vi "HFRR ADV v05 new software.vi"() -> ()   [LabVIEW 2025] (continued)
                  n3128 = property on="Air Temperature  ( °C )" class="XYGraph (strict)"("Y Scale.Name Label.Text"=w4162) -> ()  [unwired: 2 in, 2 out]
                }
                frame 82 {
                  n3129 = local write "S 84"(w4163) -> ()
                }
                frame 83 {
                  n3130 = local write "S 85"(w4164) -> ()
                }
                frame 84 {
                  n3131 = local write "S 86"(w4165) -> ()
                }
                frame 85 {
                  n3132 = local write "S 87"(w4166) -> ()
                }
                frame 86 {
                  n3133 = local write "S 88"(w4167) -> ()
                }
                frame 87 {
                }
                frame 88 {
                  n3134 = local write "S 90"(w4169) -> ()
                }
                frame 89 {
                  n3135 = local write "S 91"(w4170) -> ()
                }
                frame 90 {
                  n3136 = local write "S 92"(w4171) -> ()
                }
                frame 91 {
                  n3137 = local write "S 93"(w4172) -> ()
                }
                frame 92 {
                  n3138 = local write "S 94"(w4173) -> ()
                }
                frame 93 {
                  n3139 = local write "S 95"(w4174) -> ()
                }
                frame 94 {
                  n3140 = local write "S 96"(w4175) -> ()
                }
                frame 95 {
                  n3141 = local write "S 97"(w4176) -> ()
                }
                frame 96 {
                  n3142 = local write "S 98"(w4177) -> ()
                }
                frame 97 {
                  n3143 = local write "S 99"(w4178) -> ()
                }
                frame 98 {
                  n3144 = local write "S 100"(w4179) -> ()
                }
                frame 99 {
                  n3145 = local write "S 101"(w4180) -> ()
                }
                frame 100 {
                  n3146 = local write "S 102"(w4181) -> ()
                }
                frame 101 {
                  n3147 = local write "S 103"(w4182) -> ()
                }
                frame 102 {
                  n3148 = local write "S 104"(w4183) -> ()
                }
                frame 103 {
                  n3149 = local write "S 105"(w4184) -> ()
                }
                frame 104 {
                  n3150 = local write "S 106"(w4185) -> ()
                }
                frame 105 {
                }
                frame 106 {
                  n3151 = property on="OK Button 17" class="Bool (strict)"("Boolean Text.Text"=w4186) -> ()  [unwired: 2 in, 2 out]
                }
                frame 107 {
                  n3152 = property on="OK Button 16" class="Bool (strict)"("Boolean Text.Text"=w4187) -> ()  [unwired: 2 in, 2 out]
                }
                frame 108 {
                  n3153 = property on="TITTLE" class="Str"("Caption.Text"=w4188) -> ()  [unwired: 2 in, 2 out]
                }
                frame 109 {
                  "String 30" <- w4189
                }
                frame 110 {
                  n3154 = property on="Test Date" class="Str"("Caption.Text"=w4190) -> ()  [unwired: 2 in, 2 out]
                  "String 31" <- w4190
                }
                frame 111 {
                  n3155 = property on="Sample ID" class="Str"("Caption.Text"=w4191) -> ()  [unwired: 2 in, 2 out]
                  "String 32" <- w4191
                }
                frame 112 {
                  n3156 = property on="Tested by" class="Str"("Caption.Text"=w4192) -> ()  [unwired: 2 in, 2 out]
                  "String 33" <- w4192
                }
                frame 113 {
                  n3157 = property on="System Configured Printers 2" class="Arr (strict)"("Caption.Text"=w4193) -> ()  [unwired: 2 in, 2 out]
                }
                frame 114 {
                  n3158 = property on="Selected Printer" class="Str"("Caption.Text"=w4194) -> ()  [unwired: 2 in, 2 out]
                }
                frame 115 {
                  n3159 = property on="Select Printer 3" class="DigNum (strict)"("Caption.Text"=w4195) -> ()  [unwired: 2 in, 2 out]
                }
                frame 116 {
                  n3160 = property on="Print" class="Bool (strict)"("Boolean Text.Text"=w4196) -> ()  [unwired: 2 in, 2 out]
                }
                frame 117 {
                  "String 41" <- w4197
                }
                frame 118 {
                  n3161 = property on="tested by" class="Str"("Caption.Text"=w4198) -> ()  [unwired: 2 in, 2 out]
                }
                frame 119 {
                }
                frame 120 {
                  n3162 = property on="Export" class="Bool (strict)"("Boolean Text.Text"=w4199) -> ()  [unwired: 2 in, 2 out]
                }
                frame 121 {
                  n3163 = property on="TEMP INTERCEPT:" class="DigNum (strict)"("Caption.Text"=w4200) -> ()  [unwired: 2 in, 2 out]
                }
                frame 122 {
                  n3164 = property on="AIR TEMP INTERCEPT:" class="DigNum (strict)"("Caption.Text"=w4201) -> ()  [unwired: 2 in, 2 out]
                }
                frame 123 {
                  n3165 = property on="Select File Type" class="Enum (strict)"("Caption.Text"=w4202) -> ()  [unwired: 2 in, 2 out]
                }
                frame 124 {
                  n3166 = property on="s.NO" class="Str"("Caption.Text"=w4203) -> ()  [unwired: 2 in, 2 out]
                  "String 45" <- w4203
                }
                frame 125 {
                  n3167 = property on="trip1 8" class="Bool (strict)"("Boolean Text.Text"=w4204) -> ()  [unwired: 2 in, 2 out]
                }
                frame 126, Default {
                }
              }
            }
          }
          frame #1 {
            w4212 = TRUE ("Visible")
            n3168 = local read "S 91"() -> (w4229:string)
            n3169 = local read "S 90"() -> (w4228:string)
            n3170 = local read "S 88"() -> (w4227:string)
            n3171 = property on="File Path" class="Path"("Caption.Text"=w4228) -> ()  [unwired: 2 in, 2 out]
            n3172 = property on="SrvM CP" class="Bool (strict)"("Boolean Text.Text"=w4227) -> ()  [unwired: 2 in, 2 out]
            n3173 = local read "S 71"() -> (w4222:string)
            n3174 = local read "S 86"() -> (w4224:string)
            n3175 = local read "S 85"() -> (w4225:string)
            n3176 = local read "S 87"() -> (w4223:string)
            n3177 = local read "S 84"() -> (w4226:string)
            n3178 = local read "S 103"() -> (w4211:string)
            n3179 = local read "S 104"() -> (w4210:string)
            n3180 = property on="ENTER THE NEW PASSWORD" class="Str"("Caption.Text"=w4223) -> ()  [unwired: 2 in, 2 out]
            n3181 = property on="Password" class="Str"("Caption.Text"=w4225) -> ()  [unwired: 2 in, 2 out]
            n3182 = property on="ENTER CURRENT PASSWORD" class="Str"("Caption.Text"=w4224) -> ()  [unwired: 2 in, 2 out]
            n3183 = property on="EDIT" class="Bool (strict)"("Boolean Text.Text"=w4222) -> ()  [unwired: 2 in, 2 out]
            n3184 = property on="SAVE" class="Bool (strict)"("Boolean Text.Text"=w4226) -> ()  [unwired: 2 in, 2 out]
            n3185 = Build Array(w4211, w4210) -> (w4209:string[])
            n3186 = property on="Heater Button" class="Bool (strict)"("Strings [4]"=w4209) -> ()  [unwired: 2 in, 2 out]
            n3187 = property on="CH-HUMIDITY WET" class="DigNum (strict)"("Caption.Size to Text?"=w4212) -> ()  [unwired: 2 in, 2 out]
            n3188 = property on="CH-HUMIDITY DRY" class="DigNum (strict)"("Caption.Size to Text?"=w4212) -> ()  [unwired: 2 in, 2 out]
            n3189 = property on="CH-POWER -" class="DigNum (strict)"("Caption.Size to Text?"=w4212) -> ()  [unwired: 2 in, 2 out]
            n3190 = property on="CH-HEATER" class="DigNum (strict)"("Caption.Size to Text?"=w4212) -> ()  [unwired: 2 in, 2 out]
            n3191 = property on="CH-POWER +" class="DigNum (strict)"("Caption.Size to Text?"=w4212) -> ()  [unwired: 2 in, 2 out]
            n3192 = local read "S 92"() -> (w4221:string)
            n3193 = local read "S 93"() -> (w4220:string)
            n3194 = local read "S 105"() -> (w4207:string)
            n3195 = local read "S 106"() -> (w4206:string)
            n3196 = Build Array(w4221, w4220) -> ()  [unwired: 1 out]
            n3197 = Build Array(w4207, w4206) -> (w4208:string[])
            n3198 = local read "S 95"() -> (w4218:string)
            n3199 = local read "S 94"() -> (w4219:string)
            n3200 = local read "bs"() -> (w4234:string)
            n3201 = local read "as"() -> (w4235:string)
            n3202 = property on="Humidity" class="Bool (strict)"("Strings [4]"=w4208) -> ()  [unwired: 2 in, 2 out]
            n3203 = Concatenate Strings(w4234, "\r", w4235) -> ()  [unwired: 1 out]
            n3204 = property on="STROKE GAIN :" class="DigNum (strict)"("Caption.Text"=w4218) -> ()  [unwired: 2 in, 2 out]
            n3205 = property on="DISPLACEMENT :" class="DigNum (strict)"("Caption.Text"=w4219) -> ()  [unwired: 2 in, 2 out]
            n3206 = property on="Rh After" class="DigNum (strict)"("Caption.Size to Text?"=TRUE ("Caption.Size to Text")) -> ()  [unwired: 2 in, 2 out]
            n3207 = local read "S 48"() -> (w4258:string)
            n3208 = local read "S 50"() -> (w4256:string)
            n3209 = local read "S 51"() -> (w4255:string)
            n3210 = local read "S 49"() -> (w4257:string)
            n3211 = local read "S 52"() -> (w4254:string)
            n3212 = local read "as"() -> (w4239:string)
            n3213 = local read "bs"() -> (w4240:string)
            n3214 = local read "S 56"() -> (w4253:string)
            n3215 = local read "S 57"() -> (w4252:string)
            n3216 = local read "S 58"() -> (w4251:string)
            n3217 = local read "S 59"() -> (w4250:string)
            n3218 = property on="OPEN" class="Bool (strict)"("Boolean Text.Text"=w4254) -> ()  [unwired: 2 in, 2 out]
            n3219 = property on="OPEN 1" class="Bool (strict)"("Boolean Text.Text"=w4258) -> ()  [unwired: 2 in, 2 out]
            n3220 = property on="OPEN 2" class="Bool (strict)"("Boolean Text.Text"=w4257) -> ()  [unwired: 2 in, 2 out]
            n3221 = property on="OPEN 3" class="Bool (strict)"("Boolean Text.Text"=w4256) -> ()  [unwired: 2 in, 2 out]
            n3222 = property on="OPEN 4" class="Bool (strict)"("Boolean Text.Text"=w4255) -> ()  [unwired: 2 in, 2 out]
            n3223 = Concatenate Strings(w4240, "\r", w4239) -> ()  [unwired: 1 out]
            n3224 = local read "S 102"() -> (w4213:string)
            n3225 = property on="КОФ1" class="DigNum (strict)"("Caption.Text"=w4253) -> ()  [unwired: 2 in, 2 out]
            n3226 = local read "S 98"() -> (w4217:string)
            n3227 = local read "S 99"() -> (w4216:string)
            n3228 = local read "S 100"() -> (w4215:string)
            n3229 = local read "S 101"() -> (w4214:string)
            n3230 = property on="КОФ2" class="DigNum (strict)"("Caption.Text"=w4252) -> ()  [unwired: 2 in, 2 out]
            n3231 = property on="КОФ3" class="DigNum (strict)"("Caption.Text"=w4251) -> ()  [unwired: 2 in, 2 out]
            n3232 = property on="КОФ4" class="DigNum (strict)"("Caption.Text"=w4250) -> ()  [unwired: 2 in, 2 out]
            n3233 = local read "bs"() -> (w4238:string)
            n3234 = local read "as"() -> (w4237:string)
            n3235 = property on="CH-POWER +" class="DigNum (strict)"("Caption.Text"=w4217) -> ()  [unwired: 2 in, 2 out]
            n3236 = property on="CH-POWER -" class="DigNum (strict)"("Caption.Text"=w4216) -> ()  [unwired: 2 in, 2 out]
            n3237 = property on="CH-HEATER" class="DigNum (strict)"("Caption.Text"=w4215) -> ()  [unwired: 2 in, 2 out]
            n3238 = property on="CH-HUMIDITY DRY" class="DigNum (strict)"("Caption.Text"=w4214) -> ()  [unwired: 2 in, 2 out]
            n3239 = property on="CH-HUMIDITY WET" class="DigNum (strict)"("Caption.Text"=w4213) -> ()  [unwired: 2 in, 2 out]
            n3240 = local read "S 60"() -> (w4249:string)
            n3241 = local read "S 54"() -> (w4259:string)
            n3242 = Concatenate Strings(w4238, "\r", w4237) -> ()  [unwired: 1 out]
            n3243 = Concatenate Strings(w4259, w4249) -> ()  [unwired: 1 out]
            n3244 = local read "S 77"() -> (→"String 43":string)
            n3245 = local read "S 76"() -> (w4232:string)
            n3246 = local read "S 78"() -> (w4231:string)
            n3247 = local read "S 71"() -> (w4243:string)
            n3248 = local read "S 66"() -> (w4248:string)
            n3249 = local read "S 67"() -> (w4247:string)
            n3250 = local read "S 68"() -> (w4246:string)
            n3251 = local read "S 69"() -> (w4245:string)
            n3252 = local read "S 70"() -> (w4244:string)
            n3253 = property on="AIR TEMP" class="DigNum (strict)"("Caption.Text"=w4231) -> ()  [unwired: 2 in, 2 out]
            n3254 = property on="Set Strk" class="DigNum (strict)"("Caption.Text"=w4232) -> ()  [unwired: 2 in, 2 out]
            n3255 = property on="FRIC. FORCE :" class="DigNum (strict)"("Caption.Text"=w4248) -> ()  [unwired: 2 in, 2 out]
            n3256 = property on="TEMPERATURE :" class="DigNum (strict)"("Caption.Text"=w4247) -> ()  [unwired: 2 in, 2 out]
            n3257 = property on="SPEED OUT:" class="DigNum (strict)"("Caption.Text"=w4246) -> ()  [unwired: 2 in, 2 out]
            n3258 = property on="AIR TEMPERATURE :" class="DigNum (strict)"("Caption.Text"=w4245) -> ()  [unwired: 2 in, 2 out]
            n3259 = property on="HUMIDITY:" class="DigNum (strict)"("Caption.Text"=w4244) -> ()  [unwired: 2 in, 2 out]
            n3260 = property on="EDIT" class="Bool (strict)"("Boolean Text.Text"=w4243) -> ()  [unwired: 2 in, 2 out]
            n3261 = local read "S 79"() -> (w4230:string)
          }
          frame #2 {
          }
        }
        n3262 = local write "Lan flag"(10.0 ("Lan flag")) -> ()
      }
      frame Enabled {
      }
    }
    n3263 = Wait (ms)(milliseconds to wait=u32 2000) -> ()  [unwired: 1 out]
    n3264 = local read "Quit"() -> (w4033:bool)
  }
  n3265 = disable-structure shown="Disabled" {
    frame Disabled {
      n3266 = while {
        tunnel: [w4261] -> _
        i -> [w4261]
        stop <- w4260 continue-if-true
        n3267 = Wait (ms)(milliseconds to wait=u32 50) -> ()  [unwired: 1 out]
        n3268 = stacked-sequence {
          frame #0 {
            # "Controls Text color"
            # "Controls BG color"
            n3269 = property on="FILE" class="Str"("Text.Text Colors:Text Color"="SC  Text") -> ()  [unwired: 2 in, 2 out]
            n3270 = property on="Fuel Discription :" class="Str"("Text.Text Colors:Text Color"="SC  Text") -> ()  [unwired: 2 in, 2 out]
            n3271 = property on="tested by" class="Str"("Text.Text Colors:Text Color"="SC  Text") -> ()  [unwired: 2 in, 2 out]
            n3272 = property on="Remarks :" class="Str"("Text.Text Colors:Text Color"="SC  Text") -> ()  [unwired: 2 in, 2 out]
            n3273 = property class="DigNum (strict)"("Numeric Text.Text Colors:BG Color"="NC BG") -> ()  [unwired: 2 in, 2 out]
            n3274 = property class="DigNum (strict)"("Numeric Text.Text Colors:BG Color"="NC BG") -> ()  [unwired: 2 in, 2 out]
            n3275 = property class="DigNum (strict)"("Numeric Text.Text Colors:BG Color"="NC BG") -> ()  [unwired: 2 in, 2 out]
            n3276 = property class="DigNum (strict)"("Numeric Text.Text Colors:BG Color"="NC BG") -> ()  [unwired: 2 in, 2 out]
            n3277 = property class="DigNum (strict)"("Numeric Text.Text Colors:BG Color"="NC BG") -> ()  [unwired: 2 in, 2 out]
            n3278 = property class="DigNum (strict)"("Numeric Text.Text Colors:BG Color"="NC BG") -> ()  [unwired: 2 in, 2 out]
            n3279 = property class="DigNum (strict)"("Numeric Text.Text Colors:BG Color"="NC BG") -> ()  [unwired: 2 in, 2 out]
            n3280 = property class="DigNum (strict)"("Numeric Text.Text Colors:BG Color"="NC BG") -> ()  [unwired: 2 in, 2 out]
            n3281 = property class="DigNum (strict)"("Numeric Text.Text Colors:BG Color"="NC BG") -> ()  [unwired: 2 in, 2 out]
            n3282 = property class="DigNum (strict)"("Numeric Text.Text Colors:BG Color"="NC BG") -> ()  [unwired: 2 in, 2 out]
            n3283 = property class="DigNum (strict)"("Numeric Text.Text Colors:BG Color"="NC BG") -> ()  [unwired: 2 in, 2 out]
            n3284 = property class="DigNum (strict)"("Numeric Text.Text Colors:BG Color"="NC BG") -> ()  [unwired: 2 in, 2 out]
            n3285 = property on="FILE" class="Str"("Text.Text Colors:BG Color"="SC BG 3") -> ()  [unwired: 2 in, 2 out]
            n3286 = property on="Fuel Discription :" class="Str"("Text.Text Colors:BG Color"="SC BG 3") -> ()  [unwired: 2 in, 2 out]
            n3287 = property on="tested by" class="Str"("Text.Text Colors:BG Color"="SC BG 3") -> ()  [unwired: 2 in, 2 out]
            n3288 = property on="Remarks :" class="Str"("Text.Text Colors:BG Color"="SC BG 3") -> ()  [unwired: 2 in, 2 out]
            n3289 = property class="DigNum (strict)"("Numeric Text.Text Colors:Text Color"="NC Text") -> ()  [unwired: 2 in, 2 out]
            n3290 = property class="DigNum (strict)"("Numeric Text.Text Colors:Text Color"="NC Text") -> ()  [unwired: 2 in, 2 out]
            n3291 = property class="DigNum (strict)"("Numeric Text.Text Colors:Text Color"="NC Text") -> ()  [unwired: 2 in, 2 out]
            n3292 = property class="DigNum (strict)"("Numeric Text.Text Colors:Text Color"="NC Text") -> ()  [unwired: 2 in, 2 out]
            n3293 = property class="DigNum (strict)"("Numeric Text.Text Colors:Text Color"="NC Text") -> ()  [unwired: 2 in, 2 out]
            n3294 = property class="DigNum (strict)"("Numeric Text.Text Colors:Text Color"="NC Text") -> ()  [unwired: 2 in, 2 out]
            n3295 = property class="DigNum (strict)"("Numeric Text.Text Colors:Text Color"="NC Text") -> ()  [unwired: 2 in, 2 out]
            n3296 = property class="DigNum (strict)"("Numeric Text.Text Colors:Text Color"="NC Text") -> ()  [unwired: 2 in, 2 out]
            n3297 = property class="DigNum (strict)"("Numeric Text.Text Colors:Text Color"="NC Text") -> ()  [unwired: 2 in, 2 out]
            n3298 = property class="DigNum (strict)"("Numeric Text.Text Colors:Text Color"="NC Text") -> ()  [unwired: 2 in, 2 out]
            n3299 = property class="DigNum (strict)"("Numeric Text.Text Colors:Text Color"="NC Text") -> ()  [unwired: 2 in, 2 out]
            n3300 = property class="DigNum (strict)"("Numeric Text.Text Colors:Text Color"="NC Text") -> ()  [unwired: 2 in, 2 out]
            n3301 = property class="DigNum (strict)"("Numeric Text.Text Colors:Text Color"="NI Text  2") -> ()  [unwired: 2 in, 2 out]
            n3302 = property class="DigNum (strict)"("Numeric Text.Text Colors:Text Color"="NI Text  2") -> ()  [unwired: 2 in, 2 out]
            n3303 = property class="DigNum (strict)"("Numeric Text.Text Colors:Text Color"="NI Text  2") -> ()  [unwired: 2 in, 2 out]
            n3304 = property class="DigNum (strict)"("Numeric Text.Text Colors:Text Color"="NI Text  2") -> ()  [unwired: 2 in, 2 out]
            n3305 = property class="DigNum (strict)"("Numeric Text.Text Colors:Text Color"="NI Text  2") -> ()  [unwired: 2 in, 2 out]
            n3306 = property class="DigNum (strict)"("Numeric Text.Text Colors:Text Color"="NI Text  2") -> ()  [unwired: 2 in, 2 out]
            n3307 = property class="DigNum (strict)"("Numeric Text.Text Colors:Text Color"="NI Text  2") -> ()  [unwired: 2 in, 2 out]
            n3308 = property class="DigNum (strict)"("Numeric Text.Text Colors:Text Color"="NI Text  2") -> ()  [unwired: 2 in, 2 out]
            n3309 = property class="DigNum (strict)"("Numeric Text.Text Colors:Text Color"="NI Text  2") -> ()  [unwired: 2 in, 2 out]
            n3310 = property class="DigNum (strict)"("Numeric Text.Text Colors:Text Color"="NI Text  2") -> ()  [unwired: 2 in, 2 out]
            n3311 = property class="DigNum (strict)"("Numeric Text.Text Colors:Text Color"="NI Text  2") -> ()  [unwired: 2 in, 2 out]
            n3312 = property class="DigNum (strict)"("Numeric Text.Text Colors:Text Color"="NI Text  2") -> ()  [unwired: 2 in, 2 out]
            n3313 = property class="DigNum (strict)"("Numeric Text.Text Colors:Text Color"="NI Text  2") -> ()  [unwired: 2 in, 2 out]
            n3314 = property class="DigNum (strict)"("Numeric Text.Text Colors:Text Color"="NI Text  2") -> ()  [unwired: 2 in, 2 out]
            n3315 = property class="DigNum (strict)"("Numeric Text.Text Colors:Text Color"="NI Text  2") -> ()  [unwired: 2 in, 2 out]
            n3316 = property on="Coefficient Of Friction" class="XYGraph (strict)"("Plot Area:Colors:FG Color"="GFG  2", "Plot Area:Colors:BG Color"="GBG   2") -> ()  [unwired: 2 in, 2 out]
            n3317 = property on="Humidity ( %RH )" class="XYGraph (strict)"("Plot Area:Colors:FG Color"="GFG  2", "Plot Area:Colors:BG Color"="GBG   2") -> ()  [unwired: 2 in, 2 out]
            n3318 = property on="Air Temperature  ( °C )" class="XYGraph (strict)"("Plot Area:Colors:FG Color"="GFG  2", "Plot Area:Colors:BG Color"="GBG   2") -> ()  [unwired: 2 in, 2 out]
            n3319 = property on="Sample Temperature ( °C )" class="XYGraph (strict)"("Plot Area:Colors:FG Color"="GFG  2", "Plot Area:Colors:BG Color"="GBG   2") -> ()  [unwired: 2 in, 2 out]
            n3320 = property class="DigNum (strict)"("Numeric Text.Text Colors:BG Color"="NI BG 2") -> ()  [unwired: 2 in, 2 out]
            n3321 = property class="DigNum (strict)"("Numeric Text.Text Colors:BG Color"="NI BG 2") -> ()  [unwired: 2 in, 2 out]
            n3322 = property class="DigNum (strict)"("Numeric Text.Text Colors:BG Color"="NI BG 2") -> ()  [unwired: 2 in, 2 out]
            n3323 = property class="DigNum (strict)"("Numeric Text.Text Colors:BG Color"="NI BG 2") -> ()  [unwired: 2 in, 2 out]
            n3324 = property class="DigNum (strict)"("Numeric Text.Text Colors:BG Color"="NI BG 2") -> ()  [unwired: 2 in, 2 out]
            n3325 = property class="DigNum (strict)"("Numeric Text.Text Colors:BG Color"="NI BG 2") -> ()  [unwired: 2 in, 2 out]
            n3326 = property class="DigNum (strict)"("Numeric Text.Text Colors:BG Color"="NI BG 2") -> ()  [unwired: 2 in, 2 out]
            n3327 = property class="DigNum (strict)"("Numeric Text.Text Colors:BG Color"="NI BG 2") -> ()  [unwired: 2 in, 2 out]
            n3328 = property class="DigNum (strict)"("Numeric Text.Text Colors:BG Color"="NI BG 2") -> ()  [unwired: 2 in, 2 out]
            n3329 = property class="DigNum (strict)"("Numeric Text.Text Colors:BG Color"="NI BG 2") -> ()  [unwired: 2 in, 2 out]
            n3330 = property class="DigNum (strict)"("Numeric Text.Text Colors:BG Color"="NI BG 2") -> ()  [unwired: 2 in, 2 out]
            n3331 = property class="DigNum (strict)"("Numeric Text.Text Colors:BG Color"="NI BG 2") -> ()  [unwired: 2 in, 2 out]
            n3332 = property class="DigNum (strict)"("Numeric Text.Text Colors:BG Color"="NI BG 2") -> ()  [unwired: 2 in, 2 out]
            n3333 = property class="DigNum (strict)"("Numeric Text.Text Colors:BG Color"="NI BG 2") -> ()  [unwired: 2 in, 2 out]
            n3334 = property class="DigNum (strict)"("Numeric Text.Text Colors:BG Color"="NI BG 2") -> ()  [unwired: 2 in, 2 out]
            n3335 = property class="Bool"("Colors [4]"="Boolean BC T & BG") -> ()  [unwired: 2 in, 2 out]
            n3336 = property on="Save & Continue" class="Bool (strict)"("Colors [4]"="Boolean BC T & BG") -> ()  [unwired: 2 in, 2 out]
            n3337 = property on="Heater Button" class="Bool (strict)"("Colors [4]"="Boolean BC T & BG") -> ()  [unwired: 2 in, 2 out]
            n3338 = property class="Bool"("Colors [4]"="Boolean BC T & BG") -> ()  [unwired: 2 in, 2 out]
            n3339 = property on="Humidity" class="Bool (strict)"("Colors [4]"="Boolean BC T & BG") -> ()  [unwired: 2 in, 2 out]
            n3340 = property class="Bool (strict)"("Colors [4]"="Boolean BC T & BG") -> ()  [unwired: 2 in, 2 out]
            n3341 = property on="RUN" class="Bool (strict)"("Colors [4]"="Boolean BC T & BG") -> ()  [unwired: 2 in, 2 out]
            n3342 = property on="trip1 8" class="Bool (strict)"("Colors [4]"="Boolean BC T & BG") -> ()  [unwired: 2 in, 2 out]
            n3343 = property class="Bool"("Colors [4]"="Boolean BC T & BG") -> ()  [unwired: 2 in, 2 out]
            n3344 = property class="Bool (strict)"("Colors [4]"="Boolean BC T & BG") -> ()  [unwired: 2 in, 2 out]
            n3345 = property on="OPEN 1" class="Bool (strict)"("Colors [4]"="Boolean BC T & BG 2") -> ()  [unwired: 2 in, 2 out]
            n3346 = property on="OPEN 2" class="Bool (strict)"("Colors [4]"="Boolean BC T & BG 2") -> ()  [unwired: 2 in, 2 out]
            n3347 = property on="OPEN 3" class="Bool (strict)"("Colors [4]"="Boolean BC T & BG 2") -> ()  [unwired: 2 in, 2 out]
            n3348 = property on="OPEN 4" class="Bool (strict)"("Colors [4]"="Boolean BC T & BG 2") -> ()  [unwired: 2 in, 2 out]
            n3349 = property on="OPEN" class="Bool (strict)"("Colors [4]"="Boolean BC T & BG 2") -> ()  [unwired: 2 in, 2 out]
            n3350 = property on="rstv2" class="Bool"("Colors [4]"="Boolean BC T & BG 2") -> ()  [unwired: 2 in, 2 out]
            n3351 = property on="RST CP" class="Bool"("Colors [4]"="Boolean BC T & BG 2") -> ()  [unwired: 2 in, 2 out]
            n3352 = property on="RSTV1 3" class="Bool"("Colors [4]"="Boolean BC T & BG 2") -> ()  [unwired: 2 in, 2 out]
            n3353 = property on="RSTV1 2" class="Bool"("Colors [4]"="Boolean BC T & BG 2") -> ()  [unwired: 2 in, 2 out]
          }
          frame #1 {
          }
        }
        n3354 = local read "Quit"() -> (w4260:bool)
      }
    }
    frame Enabled {
    }
  }
  n3355 = while {
    shift-right: [w4278] -> _
    shift-left: _ -> [w4279]
    shift-right: [w4276] -> _
    shift-left: T14 {"Read Heave and Surge"="", "Bytes at Heave Port"=0.0, "Heave and Surge COM Port:"="COM9", "Com Port 2"="COM7", "Residual Due"="", "Heave COM Status 2"=TRUE, "Heave COM Status"=TRUE, "Port 2"=TRUE, "Sway PPR"=6400.0, "Surge PPR"=6400.0, "Heave PPR"=6400.0, "Sway Pitch"=2.0, "Surge Pitch"=3.0, "Heave Pitch"=4.0, "Sway Pulses/mm"=320.0, "Surge Pulses/mm"=1600.0, "Heave Pulses/mm"=1600.0, "inner loop"=0.0, "Read Heave and Surge 2"="", "String 36"="", "Write S"=FALSE, "WriteCC1"=[""], "Heave COM Loop"=0, "LastCom"="", "EXIT"=FALSE, "Error Heave"={"status"=TRUE, "code"=-1073807343, "source"=""}} -> [w4275]
    shift-right: [w4273] -> _
    shift-left: enum16{"init", "MAIN", "Panel Close"}."init" -> [w4274]
    stop <- w4277 stop-if-true
    n3356 = case shown="\"init\"" w4274 {
      tunnel: w4279 -> [w4293 w4308 w4378 w4380]
      tunnel: [w4287 w4326 w4378 w4380] -> w4278
      tunnel: [_ _ TRUE _] -> w4277
      tunnel: [w4283 w4323 w4376 w4379] -> w4276
      tunnel: w4275 -> [w4290 w4307 w4376 w4379]
      tunnel: [enum16{"init", "MAIN", "Panel Close"}."MAIN" w4301 _ _] -> w4273
      frame "init" {
        n3357 = Bundle By Name(cluster=w4290, "Heave and Surge COM Port:"="C3 :") -> (w4289:T14)
        n3358 = call "Instrument fgv.vi"("Enum"=T24."INIT", "error in (no error) 2"=w4293, "INPUT"=w4289) -> ("error"=w4291:errorcluster, "output"=w4286:T14)  [unwired: 6 in, 1 out]
        n3359 = case shown="No Error" w4291 {
          selector: w4291 -> [w4295 _]
          tunnel: [w4295 w4299] -> w4287
          tunnel: w4286 -> [w4294 w4297]
          tunnel: [w4294 w4296] -> w4284
          frame No Error {
          }
          frame Error {
            n3360 = call "Instrument fgv.vi"("Enum"=T24."ERROR INIT", "INPUT"=w4297) -> ("error"=w4300:errorcluster, "output"=w4296:T14)  [unwired: 7 in, 1 out]
            n3361 = call <vilib>:"Clear Errors.vi"("error in (no error)"=w4300) -> ("error out"=w4299:errorcluster)  [unwired: 5 in, 1 out]
          }
        }
        n3362 = local read "LastCom"() -> (w4282:string)
        n3363 = Unbundle By Name(w4284) -> ("Heave COM Status 2"=→"COM Status" →"Instrument Status":bool, "Error Heave"=→"Error":errorcluster)  [unwired: 1 out]
        n3364 = Bundle By Name(cluster=w4284, "LastCom"=w4282) -> (w4283:T14)
      }
      frame "MAIN" {
        n3365 = Unbundle By Name(w4307) -> ("Com Port 2"=w4328:refnum<visa-resource-name>)
        n3366 = local write "Com Port 4"(w4328) -> ()
        n3367 = local read "C3 :"() -> (w4305:refnum<visa-resource-name>)
        n3368 = Divide(x="Heave PPR", y="Heave Pitch") -> (x/y=→"Heave Pulses/mm":dbl)
        n3369 = Bundle By Name(cluster=w4307, "Heave and Surge COM Port:"=w4305) -> (w4306:T14)
        n3370 = Equal?(x=w4328, y=w4305) -> (x = y?=w4327:bool)
        n3371 = Divide(x="Sway PPR", y="Sway Pitch") -> (x/y=→"Sway Pulses/mm":dbl)
        n3372 = case shown="False" w4327 {
          tunnel: [w4332 w4349] -> w4326
          tunnel: w4308 -> [w4333 w4355]
          tunnel: w4306 -> [w4331 w4353]
          tunnel: [w4330 w4348] -> w4323
          frame False {
            n3373 = call <vilib>:"Clear Errors.vi"("error in (no error)"=w4333) -> ("error out"=w4329:errorcluster)  [unwired: 5 in, 1 out]
            n3374 = call "Instrument fgv.vi"("Enum"=T24."ERROR INIT", "error in (no error) 2"=w4329, "INPUT"=w4331) -> ("error"=w4335:errorcluster, "output"=w4330:T14)  [unwired: 6 in, 1 out]
            n3375 = call <vilib>:"Clear Errors.vi"("error in (no error)"=w4335) -> ("error out"=w4332:errorcluster)  [unwired: 5 in, 1 out]
          }
          frame True {
            n3376 = call "Instrument fgv.vi"("Enum"=T24."READ", "error in (no error) 2"=w4355, "INPUT"=w4353) -> ("error"=w4354:errorcluster, "output"=w4345:T14)  [unwired: 6 in, 1 out]
            n3377 = Bundle By Name(cluster=w4345, "String 36"="String 11") -> (w4344:T14)
            n3378 = case shown="True" "Write S" {
              selector: "Write S" -> [_ w4375]
              tunnel: w4354 -> [w4368 w4374]
              tunnel: [w4368 w4373] -> w4341
              tunnel: w4344 -> [w4367 w4370]
              tunnel: [w4367 w4369] -> w4340
              frame False {
              }
              frame True {
                n3379 = Not(x=w4375) -> (.not. x?=w4371:bool)
                n3380 = local write "Write S"(w4371) -> ()
                n3381 = call "Instrument fgv.vi"("Enum"=T24."MANUAL WRITE", "error in (no error) 2"=w4374, "INPUT"=w4370) -> ("error"=w4373:errorcluster, "output"=w4369:T14)  [unwired: 6 in, 1 out]
              }
            }
            n3382 = Array Size(array="WriteHumidity") -> (size(s)=w4338:i32)
            n3383 = Greater Than 0?(x=w4338) -> (x > 0?=w4336:bool)
            n3384 = call "Instrument fgv.vi"("Enum"=T24."WRITE", "error in (no error) 2"=w4341, "WriteCC1"="WriteHumidity", "INPUT"=w4340) -> ("error"=w4351:errorcluster, "WriteCC1 2"=w4339:string[], "output"=w4350:T14)  [unwired: 5 in]
            n3385 = case shown="True" w4336 {
              tunnel: w4339 -> [_ w4357]
              frame False {
              }
              frame True {
                n3386 = local write "WriteHumidity"(w4357) -> ()
              }
            }
            n3387 = case shown="Error" w4351 {
              selector: w4351 -> [w4358 w4361]
              tunnel: w4350 -> [w4359 w4366]
              tunnel: [w4359 w4365] -> w4348
              tunnel: [w4358 w4363] -> w4349
              frame No Error {
              }
              frame Error {
                n3388 = call <vilib>:"Clear Errors.vi"("error in (no error)"=w4361) -> ("error out"=w4360:errorcluster)  [unwired: 5 in, 1 out]
                n3389 = call "Instrument fgv.vi"("Enum"=T24."ERROR INIT", "error in (no error) 2"=w4360, "INPUT"=w4366) -> ("error"=w4364:errorcluster, "output"=w4365:T14)  [unwired: 6 in, 1 out]
                n3390 = call <vilib>:"Clear Errors.vi"("error in (no error)"=w4364) -> ("error out"=w4363:errorcluster)  [unwired: 5 in, 1 out]
              }
            }
            n3391 = Unbundle By Name(w4348) -> ("LastCom"=→"LastCom":string, "Read Heave and Surge"=→"Read Humidity":string)
          }
        }
        n3392 = Divide(x="Surge PPR", y="Surge Pitch") -> (x/y=→"Surge Pulses/mm":dbl)
        n3393 = Unbundle By Name(w4323) -> ("Heave COM Status 2"=w4325:bool, "Heave COM Status"=w4324:bool, "Error Heave"=w4321:errorcluster, "Bytes at Heave Port"=→"Bytes at Humidity Port":dbl)
        n3394 = Unbundle By Name(w4321) -> ("status"=→"Humidity Port":bool)
        n3395 = Not(x=w4324) -> (.not. x?=w4309:bool)
        n3396 = local write "Error"(w4321) -> ()
        n3397 = Not(x=w4325) -> (.not. x?=w4310:bool)
        n3398 = local write "Instrument Status"(w4309) -> ()
        n3399 = local write "COM Status"(w4310) -> ()
        n3400 = local read "Quit"() -> (w4302:bool)
        n3401 = Select(t=enum16{"init", "MAIN", "Panel Close"}."Panel Close", s=w4302, f=enum16{"init", "MAIN", "Panel Close"}."MAIN") -> (s? t:f=w4301:enum16{"init", "MAIN", "Panel Close"})
      }
      frame "Panel Close" {
      }
      frame Default {
      }
    }
  }
  n3402 = while {
    stop <- w4406 stop-if-true
    n3403 = local read "Read Humidity"() -> (w4387:string)
    n3404 = call <vilib>:"High Resolution Polling Wait.vi"("seconds to wait"=0.1) -> ()  [unwired: 10 in, 1 out]
    n3405 = Spreadsheet String To Array(delimiter (Tab)=",", format string="", spreadsheet string=w4387, array type (2D Dbl)=string[] []) -> (array=w4401:string[])
    n3406 = for {
      tunnel: w4401 -> [w4411] mode=indexing
      tunnel: string[] ["STATE;", "SET;", "RH;", "T;", "AMB_RH;", "AMB_T;", "PUMP;", "FAN_IN;", "FAN_OUT;", "DEHUM;", "CURRENT;", "STALL;"] -> [w4410] mode=indexing
      tunnel: [w4409] -> w4400 mode=indexing
      n3407 = Match Pattern(string=w4411, regular expression=w4410) -> (after substring=w4409:string)  [unwired: 1 in, 3 out]
    }
    n3408 = Index Array(array=w4400) -> (element #1=→"STATE :":string, element #2=→"SET :":string, element #3=w4389:string, element #4=→"T :":string, element #5=w4386:string, element #6=→"AMB_T :":string, element #7=→"PUMP :":string, element #8=→"FAN_IN :":string, element #9=→"FAN_OUT :":string, element #10=→"DEHUM :":string, element #11=→"CURRENT :":string, element #12=→"STALL :":string)  [unwired: 12 in]
    "RH :" <- w4389
    "AMB_RH :" <- w4386
    n3409 = Fract/Exp String To Number(string=w4389) -> (number=w4381:dbl)  [unwired: 3 in, 1 out]
    n3410 = Fract/Exp String To Number(string=w4386) -> (number=w4385:dbl)  [unwired: 3 in, 1 out]
    n3411 = local write "Ambient Humidity :"(w4385) -> ()
    n3412 = Equal?(x=w4381, y=0.0) -> (x = y?=w4383:bool)
    n3413 = case shown="True" w4383 {
      tunnel: [w4407 w4408] -> w4382
      tunnel: w4381 -> [w4407 _]
      frame False {
        (unwired) 0.0
        "Humidity temp" <- w4407
      }
      frame True {
        n3414 = local read "Humidity temp"() -> (w4408:dbl)
      }
    }
    "RH Numeric:" <- w4382
    n3415 = local read "Quit"() -> (w4406:bool)
  }
  n3416 = disable-structure shown="Disabled" {
    frame Disabled {
      n3417 = while {
        tunnel: [w4645] -> _
        i -> [w4645]
        stop <- w4642 stop-if-true
        n3418 = local read "powstat"() -> (w4643:bool)
        n3419 = case shown="True" w4643 {
          frame False {
          }
          frame True {
            n3420 = local read "RUN"() -> (w4646:bool)
            n3421 = case shown="True" w4646 {
              frame False {
                w4676 = 65.0 ("y")
                n3422 = local read "Set Hz"() -> (w4704:dbl)
                n3423 = local read "NORMAL LOAD"() -> (w4705:dbl)
                n3424 = Multiply(x=w4704, y=60.0) -> (x*y=w4711:dbl)
                n3425 = Multiply(x=1.2 ("y"), y=0.949) -> (x*y=w4680:dbl)
                n3426 = Multiply(x=1.2 ("y"), y=0.8166) -> (x*y=w4684:dbl)
                n3427 = Multiply(x=1.2 ("y"), y=0.851) -> (x*y=w4679:dbl)
                n3428 = local read "FF 2"() -> (w4703:dbl)
                n3429 = Absolute Value(x=w4711) -> (abs(x)=w4709:dbl)
                n3430 = case shown="13.." w4703 {
                  tunnel: [1 2 3] -> w4701
                  frame 0..10, Default {
                    # "Normal"
                  }
                  frame 11, 12 {
                  }
                  frame 13.. {
                  }
                }
                "FF STATE" <- w4701
                n3431 = local read "TEMP"() -> (w4664:dbl)
                n3432 = local read item#-1() -> (w4678)
                n3433 = Less?(x=w4678, y=w4684) -> (x < y?=w4681:bool)
                n3434 = In Range and Coerce(upper limit=w4680, x=w4678, lower limit=w4679) -> (In Range?=w4682:bool)  [unwired: 1 out]
                n3435 = case shown="3601.." w4709 {
                  tunnel: [1 2 3] -> w4707
                  frame 0..3000, Default {
                    # "Normal"
                  }
                  frame 3001..3600 {
                  }
                  frame 3601.. {
                  }
                }
                n3436 = case shown="11.." w4705 {
                  tunnel: [1 3] -> w4706
                  frame 1..10, Default {
                  }
                  frame 11.. {
                  }
                }
                "NL STATE" <- w4706
                n3437 = Multiply(x=1.2 ("y"), y=0.95) -> (x*y=w4694:dbl)
                n3438 = Multiply(x=w4676, y=0.954) -> (x*y=w4668:dbl)
                n3439 = Or(x=w4681, y=w4682) -> (x .or. y?=w4683:bool)
                n3440 = Greater Or Equal?(x=w4678, y=w4694) -> (x >= y?=w4691:bool)
                n3441 = Multiply(x=w4676, y=0.99) -> (x*y=w4665:dbl)
                n3442 = Greater Or Equal?(x=w4664, y=w4665) -> (x >= y?=w4670:bool)
                n3443 = Greater Or Equal?(x=w4664, y=w4668) -> (x >= y?=w4667:bool)
                n3444 = case shown="0, 1, Default" w4678 {
                  tunnel: [1 3] -> w4695
                  frame 0, 1, Default {
                  }
                  frame 2.. {
                  }
                }
                n3445 = case shown="True" w4691 {
                  tunnel: [1 3] -> w4696
                  frame False {
                  }
                  frame True {
                  }
                }
                n3446 = case shown="True" w4683 {
                  tunnel: [1 2] -> w4697
                  frame False {
                  }
                  frame True {
                  }
                }
                n3447 = case shown="..0" w4664 {
                  tunnel: [2 3 3 1] -> w4671
                  frame 61, 62 {
                  }
                  frame 63.. {
                  }
                  frame ..0 {
                  }
                  frame 10..60, Default {
                  }
                }
                n3448 = case shown="True" w4670 {
                  tunnel: [1 3] -> w4672
                  frame False {
                  }
                  frame True {
                  }
                }
                n3449 = Number To Decimal String(number=w4707) -> (decimal integer string=w4708:string)  [unwired: 1 in]
                n3450 = case shown="True" w4667 {
                  tunnel: [1 2] -> w4673
                  frame False {
                  }
                  frame True {
                  }
                }
                n3451 = Number To Decimal String(number=1) -> (decimal integer string=→"Air temp":string)  [unwired: 1 in]
                n3452 = Number To Decimal String(number=w4701) -> (decimal integer string=→"ff_st":string)  [unwired: 1 in]
                n3453 = local write "sp_st"(w4708) -> ()
                n3454 = Number To Decimal String(number=w4706) -> (decimal integer string=→"nl_st":string)  [unwired: 1 in]
                n3455 = Build Array(w4671, w4672, w4673) -> (w4674:i32[])
                n3456 = Build Array(w4695, w4696, w4697) -> (w4698:i32[])
                n3457 = Array Max & Min(array=w4674) -> (max value=w4675:i32)  [unwired: 3 out]
                n3458 = Array Max & Min(array=w4698) -> (max value=w4699:i32)  [unwired: 3 out]
                n3459 = Number To Decimal String(number=w4675) -> (decimal integer string=w4663:string)  [unwired: 1 in]
                n3460 = Number To Decimal String(number=w4699) -> (decimal integer string=→"Stroke Ln 2":string)  [unwired: 1 in]
                n3461 = local write "temp_st"(w4663) -> ()
              }
              frame True {
                w4761 = 65.0 ("y")
                # "Healthy -1\nWarning -2\nError -3"
                n3462 = local read "TEMP"() -> (w4772:dbl)
                n3463 = local read "NORMAL LOAD"() -> (w4776:dbl)
                n3464 = local read "Set Hz"() -> (w4774:dbl)
                n3465 = Multiply(x=1.2 ("y"), y=0.949) -> (x*y=w4756:dbl)
                n3466 = Multiply(x=1.2 ("y"), y=0.8166) -> (x*y=w4752:dbl)
                n3467 = Multiply(x=1.2 ("y"), y=0.851) -> (x*y=w4757:dbl)
                n3468 = Multiply(x=w4761, y=0.954) -> (x*y=w4768:dbl)
                n3469 = Multiply(x=w4761, y=0.99) -> (x*y=w4771:dbl)
                n3470 = Greater Or Equal?(x=w4772, y=w4771) -> (x >= y?=w4766:bool)
                n3471 = Multiply(x=w4774, y=60.0) -> (x*y=w4780:dbl)
                n3472 = Greater Or Equal?(x=w4772, y=w4768) -> (x >= y?=w4769:bool)
                n3473 = local read "FF 2"() -> (w4775:dbl)
                n3474 = local read item#-1() -> (w4758)
                n3475 = Less?(x=w4758, y=w4752) -> (x < y?=w4755:bool)
                n3476 = In Range and Coerce(upper limit=w4756, x=w4758, lower limit=w4757) -> (In Range?=w4754:bool)  [unwired: 1 out]
                n3477 = Absolute Value(x=w4780) -> (abs(x)=w4778:dbl)
                n3478 = case shown="63.." w4772 {
                  tunnel: [2 3 3 1] -> w4765
                  frame 61, 62 {
                  }
                  frame 63.. {
                  }
                  frame ..0 {
                  }
                  frame 10..60, Default {
                  }
                }
                n3479 = case shown="True" w4766 {
                  tunnel: [1 3] -> w4764
                  frame False {
                  }
                  frame True {
                  }
                }
                n3480 = case shown="True" w4769 {
                  tunnel: [1 2] -> w4763
                  frame False {
                  }
                  frame True {
                  }
                }
                n3481 = Multiply(x=1.2 ("y"), y=0.95) -> (x*y=w4742:dbl)
                n3482 = case shown="1..10, Default" w4776 {
                  tunnel: [1 3] -> w4783
                  frame 1..10, Default {
                  }
                  frame 11.. {
                  }
                }
                n3483 = case shown="0..10, Default" w4775 {
                  tunnel: [1 2 3] -> w4782
                  frame 0..10, Default {
                  }
                  frame 11, 12 {
                  }
                  frame 13.. {
                  }
                }
                n3484 = case shown="3601.." w4778 {
                  tunnel: [1 2 3] -> w4777
                  frame 0..3000, Default {
                    # "Normal"
                  }
                  frame 3001..3600 {
                  }
                  frame 3601.. {
                  }
                }
                n3485 = Or(x=w4755, y=w4754) -> (x .or. y?=w4753:bool)
                n3486 = Greater Or Equal?(x=w4758, y=w4742) -> (x >= y?=w4745:bool)
                n3487 = case shown="0, 1, Default" w4758 {
                  tunnel: [1 3] -> w4741
                  frame 0, 1, Default {
                  }
                  frame 2.. {
                  }
                }
                n3488 = case shown="True" w4745 {
                  tunnel: [1 3] -> w4740
                  frame False {
                  }
                  frame True {
                  }
                }
                n3489 = case shown="True" w4753 {
                  tunnel: [1 2] -> w4739
                  frame False {
                  }
                  frame True {
                  }
                }
                n3490 = Build Array(w4765, w4764, w4763) -> (w4762:i32[])
                n3491 = Number To Decimal String(number=w4777) -> (decimal integer string=→"sp_st":string)  [unwired: 1 in]
                n3492 = Array Max & Min(array=w4762) -> (max value=w4759:i32)  [unwired: 3 out]
                "TEMP STATE" <- w4759
                n3493 = Number To Decimal String(number=w4783) -> (decimal integer string=w4786:string)  [unwired: 1 in]
                n3494 = Number To Decimal String(number=w4782) -> (decimal integer string=w4784:string)  [unwired: 1 in]
                n3495 = Number To Decimal String(number=w4759) -> (decimal integer string=→"temp_st":string)  [unwired: 1 in]
                n3496 = Build Array(w4741, w4740, w4739) -> (w4738:i32[])
                n3497 = local write "nl_st"(w4786) -> ()
                n3498 = local write "ff_st"(w4784) -> ()
                n3499 = Number To Decimal String(number=1) -> (decimal integer string=w4781:string)  [unwired: 1 in]
                n3500 = Array Max & Min(array=w4738) -> (max value=w4737:i32)  [unwired: 3 out]
                n3501 = local write "Air temp"(w4781) -> ()
                n3502 = Number To Decimal String(number=w4737) -> (decimal integer string=w4736:string)  [unwired: 1 in]
                n3503 = local write "Stroke Ln 2"(w4736) -> ()
              }
            }
            n3504 = local read "Stroke Ln 2"() -> (w4648:string)
            n3505 = local read "nl_st"() -> (w4654:string)
            n3506 = local read "ff_st"() -> (w4651:string)
            n3507 = local read "sp_st"() -> (w4652:string)
            n3508 = local read "temp_st"() -> (w4653:string)
            n3509 = local read "Air temp"() -> (w4647:string)
            n3510 = Replace Array Subset(array="in", new element #1=w4654, index #1=1 ("index"), new element #2=w4651, index #2=2 ("index"), new element #3=w4653, index #3=3 ("index"), new element #4=w4652, index #4=4 ("index"), new element #5=w4648, index #5=5 ("index"), new element #6=w4647, index #6=6 ("index"), new element #7="Sensor State" ("new element/subarray"), index #7=0 ("index")) -> (→"out":string[])
          }
        }
        n3511 = Wait (ms)(milliseconds to wait=u32 10) -> ()  [unwired: 1 out]
        n3512 = local read "Quit"() -> (w4642:bool)
      }
      n3513 = while {
        stop <- w4617 stop-if-true
        n3514 = local read "run replace"() -> (w4619:bool)
        n3515 = Wait (ms)(milliseconds to wait=u32 100) -> ()  [unwired: 1 out]
        n3516 = Equal?(x="FLAG 2", y=0.0) -> (x = y?=w4620:bool)
        n3517 = case shown="True" w4620 {
          frame False {
          }
          frame True {
            n3518 = local write "FLAG 2"(100.0 ("FLAG 2")) -> ()
            n3519 = call <vilib>:"Read Characters From File.vi"("file path (dialog if empty)"=path "C:/LAB-IQ-NXT/WO 2449 TT.sig", "convert eol? (no:F)"=FALSE ("append to file? (new file:F)")) -> ("character string"=w4623:string)  [unwired: 4 in, 3 out]
            n3520 = call <vilib>:"Read Characters From File.vi"("file path (dialog if empty)"=path "C:/LAB-IQ-NXT/WO 2449 TRH.sig", "convert eol? (no:F)"=FALSE ("append to file? (new file:F)")) -> ("character string"=w4624:string)  [unwired: 4 in, 3 out]
            n3521 = Decimal String To Number(string=w4623) -> (number=w4625:i32)  [unwired: 2 in, 1 out]
            n3522 = local write "Total No. of Tests"(w4625) -> ()
            n3523 = Decimal String To Number(string=w4624) -> (number=w4628:i32)  [unwired: 2 in, 1 out]
            n3524 = local write "SEN.RUN HRS"(w4628) -> ()
          }
        }
        n3525 = case shown="True" w4619 {
          frame False {
          }
          frame True {
            n3526 = Equal?(x="FLAG 4", y=0.0) -> (x = y?=w4632:bool)
            n3527 = case shown="False" w4632 {
              frame False {
                n3528 = Get Date/Time In Seconds() -> (seconds since 1Jan1904=w4638:timestamp)
                n3529 = local read "START 3"() -> (w4636:dbl)
                n3530 = To Double Precision Float(number=w4638) -> (double precision float=w4637:dbl)
                n3531 = Subtract(x=w4637, y=w4636) -> (x-y=→"SENSOR TIME":dbl)
              }
              frame True {
                n3532 = Get Date/Time In Seconds() -> (seconds since 1Jan1904=w4640:timestamp)
                n3533 = local write "FLAG 4"(100.0 ("FLAG")) -> ()
                n3534 = To Double Precision Float(number=w4640) -> (double precision float=→"START 3":dbl)
              }
            }
          }
        }
        n3535 = local read "Quit"() -> (w4617:bool)
      }
      n3536 = while {
        shift-right: [w4417] -> _
        shift-left: _ -> [w4418]
        tunnel: [w4413] -> _
        i -> [w4413]
        stop <- w4412 stop-if-true
        n3537 = Wait (ms)(milliseconds to wait=u32 50 ("Refresh Rate (ms)")) -> ()  [unwired: 1 out]
        n3538 = local read "Json End Flg"() -> (w4414:bool)
        n3539 = Not(x="Upld AR 2") -> ()  [unwired: 1 out]
        n3540 = local read "Upld AR 2"() -> (w4415:bool)
        n3541 = call "Elapsed Time9"("Time Target (s)"="Sen.Upload Rate (s)", "Reset"=FALSE, "Auto Reset"=TRUE) -> ("Time has Elapsed"=w4424:bool)  [unwired: 9 in, 7 out]
        n3542 = Or(x=w4424, y=w4414) -> (x .or. y?=w4420:bool)
        n3543 = case shown="True" w4420 {
          frame False {
          }
          frame True {
            w4516 = "\"SensorName\":\"" ("string")
            w4486 = " \"},{"
            w4511 = "\",\"SensorState\":\""
            w4513 = "\",\"SensorModelNumber\":\"" ("string")
            w4512 = "\",\"SensorRuntimeHours\":\"" ("string")
            n3544 = local read "model num"() -> (w4510:string[])
            n3545 = local read "Sensor name"() -> (w4529:string[])
            n3546 = local read "run"() -> (w4500:string[])
            n3547 = local read "SENSOR TIME"() -> (w4456:dbl)
            n3548 = local read "out"() -> (w4449:string[])
            n3549 = local read "Total No. of Tests"() -> (w4454:dbl)
            n3550 = Select(t=60.0, s="Run test 3", f=3600.0) -> (s? t:f=w4464:dbl)
            n3551 = Index Array(array=w4510, index #1=1 ("index")) -> (element #1=w4509:string, element #2=w4508:string, element #3=w4507:string, element #4=w4506:string, element #5=w4505:string, element #6=w4504:string)  [unwired: 5 in]
            n3552 = Index Array(array=w4500, index #1=1 ("index")) -> (element #1=w4499:string, element #2=w4498:string, element #3=w4497:string, element #4=w4496:string, element #5=w4495:string, element #6=w4494:string)  [unwired: 5 in]
            n3553 = Index Array(array=w4529, index #1=1 ("index")) -> (element #1=w4528:string, element #2=w4527:string, element #3=w4526:string, element #4=w4525:string, element #5=w4515:string, element #6=w4514:string)  [unwired: 5 in]
            n3554 = Index Array(array=w4449, index #1=1 ("index")) -> (element #1=w4481:string, element #2=w4480:string, element #3=w4479:string, element #4=w4478:string, element #5=w4477:string, element #6=w4476:string)  [unwired: 5 in]
            n3555 = local read "SEN.RUN HRS"() -> (w4452:dbl)
            n3556 = Divide(x=w4456, y=w4464) -> (x/y=w4463:dbl)
            n3557 = Increment(x=w4463) -> (x+1=w4459:dbl)
            n3558 = Number To Decimal String(number=w4459) -> (decimal integer string=→"run hrs":string)  [unwired: 1 in]
            n3559 = Divide(x=w4452, y=3600.0 ("f")) -> (x/y=w4447:dbl)
            n3560 = Round To Nearest(number=w4447) -> (nearest integer value=w4445:dbl)
            n3561 = Number To Decimal String(number=w4445) -> (decimal integer string=w4446:string)  [unwired: 1 in]
            n3562 = Number To Decimal String(number=w4454) -> (decimal integer string=w4455:string)  [unwired: 1 in]
            n3563 = local read "Model No"() -> (w4460:string)
            n3564 = local read "UUID"() -> (w4555:string)
            n3565 = local read "Serial No"() -> (w4559:string)
            n3566 = local read "Secret Key"() -> (w4560:string)
            n3567 = Concatenate Strings("\",\"MachineSerialNumber\":\"" ("string"), w4559) -> (w4563:string)
            n3568 = Concatenate Strings("\",\"ModelNumber\":\"" ("string"), w4460) -> (w4461:string)
            n3569 = Concatenate Strings("\",\"MachineRuntimeHours\":\"" ("string"), w4446) -> (w4564:string)
            n3570 = Concatenate Strings("\",\"MachineRuntimeCycles\":\"", w4455) -> (w4557:string)
            n3571 = Concatenate Strings(w4513, w4509) -> (w4543:string)
            n3572 = Concatenate Strings(w4512, w4499) -> (w4544:string)
            n3573 = Concatenate Strings(w4511, w4481) -> (w4542:string)
            n3574 = Concatenate Strings(w4563, w4461, w4564, w4557) -> (w4566:string)
            n3575 = Concatenate Strings(w4513, w4508) -> (w4540:string)
            n3576 = Concatenate Strings(w4512, w4498) -> (w4539:string)
            n3577 = Concatenate Strings(w4511, w4480) -> (w4541:string)
            n3578 = Concatenate Strings(w4513, w4507) -> (w4535:string)
            n3579 = Concatenate Strings(w4512, w4497) -> (w4536:string)
            n3580 = Concatenate Strings(w4511, w4479) -> (w4534:string)
            n3581 = Concatenate Strings(w4513, w4506) -> (w4532:string)
            n3582 = Concatenate Strings(w4512, w4496) -> (w4531:string)
            n3583 = Concatenate Strings(w4511, w4478) -> (w4533:string)
            n3584 = Concatenate Strings(w4543, w4544, w4542) -> (w4545:string)
            n3585 = Concatenate Strings(w4513, w4505) -> (w4522:string)
            n3586 = Concatenate Strings(w4512, w4495) -> (w4523:string)
            n3587 = Concatenate Strings(w4513, w4504) -> (w4519:string)
            n3588 = Concatenate Strings(w4512, w4494) -> (w4518:string)
            n3589 = Concatenate Strings(w4511, w4477) -> (w4521:string)
            n3590 = Concatenate Strings(w4511, w4476) -> (w4520:string)
            n3591 = Concatenate Strings("{\"SecretKey\":\"", w4560, w4566, "\",\"UUID\" : \"", w4555, "\",\"SensorInformation\":", "[{" ("string")) -> (w4493:string)
            n3592 = Concatenate Strings(w4540, w4539, w4541) -> (w4538:string)
            n3593 = Concatenate Strings(w4535, w4536, w4534) -> (w4537:string)
            n3594 = Concatenate Strings(w4532, w4531, w4533) -> (w4530:string)
            n3595 = Concatenate Strings(w4522, w4523, w4521) -> (w4524:string)
            n3596 = Concatenate Strings(w4519, w4518, w4520) -> (w4517:string)
            n3597 = Concatenate Strings(w4516, w4528, w4545, w4486) -> (w4492:string)
            n3598 = Concatenate Strings(w4516, w4527, w4538, w4486) -> (w4491:string)
            n3599 = Concatenate Strings(w4516, w4526, w4537, w4486) -> (w4490:string)
            n3600 = Concatenate Strings(w4516, w4525, w4530, w4486) -> (w4489:string)
            n3601 = Concatenate Strings(w4516, w4515, w4524, w4486) -> (w4488:string)
            n3602 = Concatenate Strings(w4516, w4514, w4517, "\"}" ("string")) -> (w4487:string)
            n3603 = Concatenate Strings(w4493, w4492, w4491, w4490, w4489, w4488, w4487, "]}" ("string")) -> (w4484:string)
            n3604 = local read "SEN.RUN HRS"() -> (w4451:dbl)
            n3605 = disable-structure shown="Disabled" {
              frame Disabled {
                n3606 = local read "state"() -> (w4570:string[])
                n3607 = Delete From Array(array=w4570, index=0) -> (array with subset deleted=w4568:string[])  [unwired: 1 in, 1 out]
                n3608 = for {
                  N: 6 -> [_]
                  tunnel: w4568 -> [w4581] mode=indexing
                  tunnel: [w4580] -> w4567 mode=indexing
                  n3609 = Equal?(x=w4581, y="Warning") -> (x = y?=w4577:bool)
                  n3610 = Equal?(x=w4581, y="Healthy") -> (x = y?=w4574:bool)
                  n3611 = Select(t="2" ("y"), s=w4577, f="3" ("y")) -> (s? t:f=w4572:string)
                  n3612 = Select(t="1" ("y"), s=w4574, f=w4572) -> (s? t:f=w4580:string)
                }
